vi "Array understanding (2).vi"() -> ()   [LabVIEW 2019]
panel:
  out "initialized array":dbl[](array[numeric])
  in  "dimension size":i32
  in  "element 2":dbl
  out "deleted portion":dbl
  out "array w/ subset deleted":dbl[](array[numeric])
  in  "index 2":i32
  out "output array":dbl[](array[numeric])
  in  "new element/subarray":dbl
  in  "index":i32
  out "element":dbl
  in  "Array":dbl[](array[numeric])
  out "size(s)":i32
  # "Array Uses and Indexing"
  # "2"
  # "1"
  # "3"
  # "4"
  # "0"
  # "5"
  # "6"
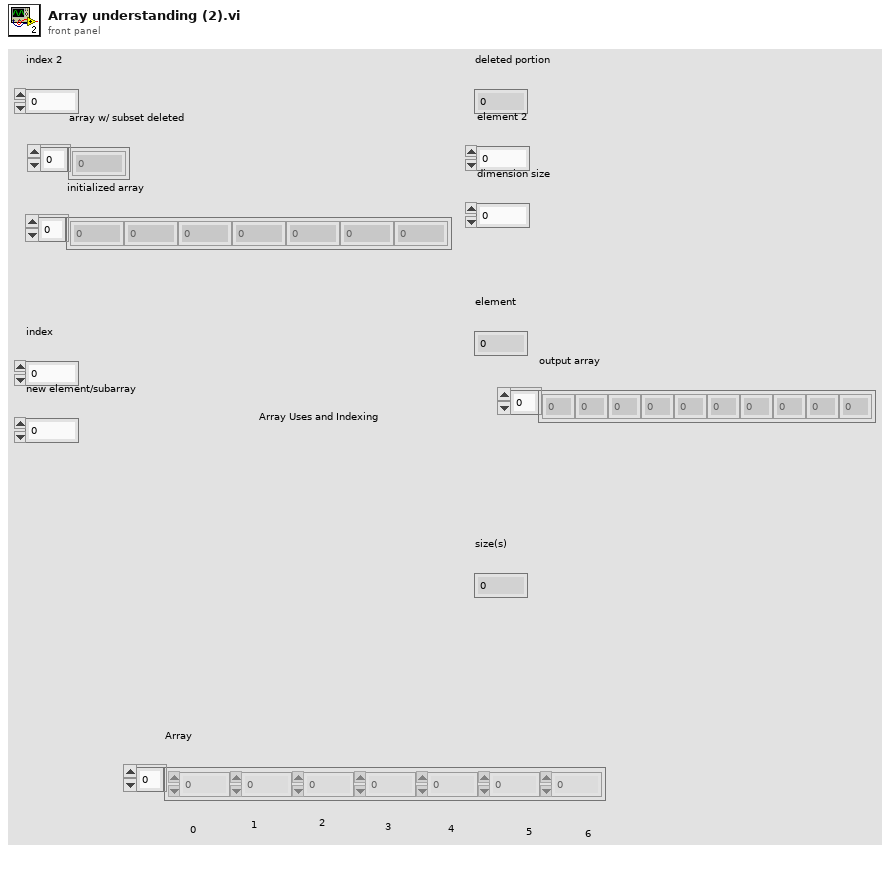
[diagram p1: front panel]
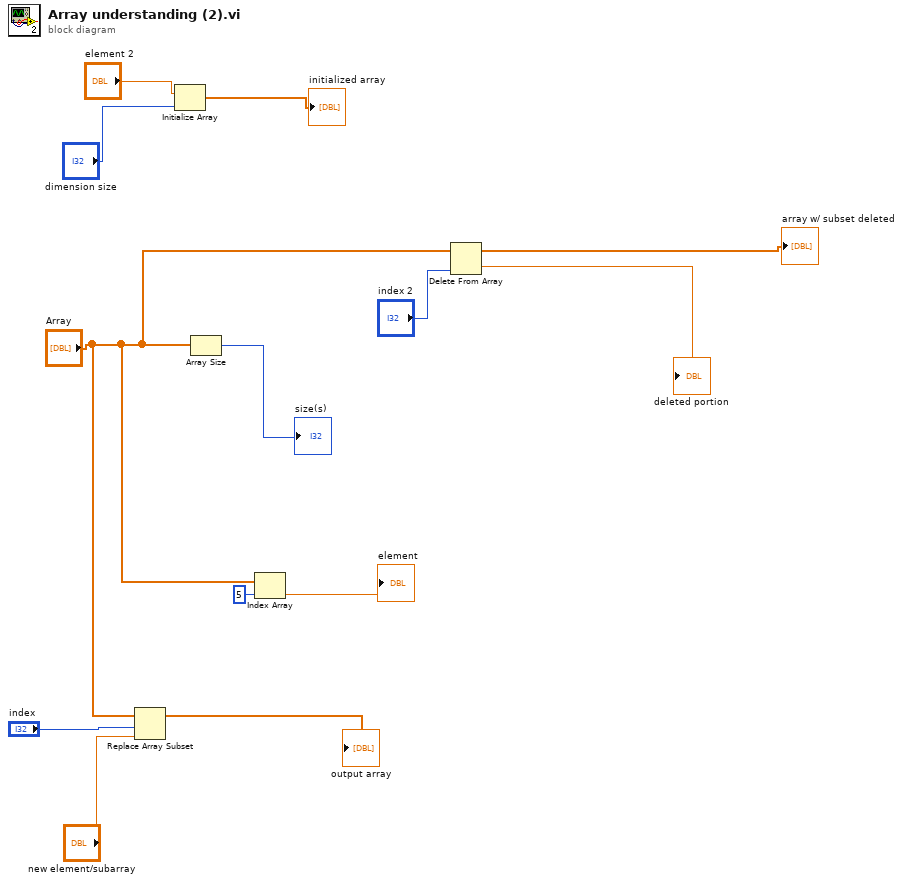
[diagram p0: block diagram]
diagram:
  n1 = Replace Array Subset "Replace Array Subset"(array="Array", new element="new element/subarray", index="index") -> (→"output array":dbl[])
  n2 = Initialize Array("element 2", "dimension size") -> (→"initialized array":dbl[])
  n3 = Array Size(array="Array") -> (size(s)=→"size(s)":i32)
  n4 = Index Array(array="Array", index=5) -> (element=→"element":dbl)
  n5 = Delete From Array "Delete From Array"(array="Array", index="index 2") -> (deleted portion=→"deleted portion":dbl, array with subset deleted=→"array w/ subset deleted":dbl[])  [unwired: 1 in]
